vi "nearCamSetExpoureTime.vi"(6 "错误输入（无错误）":errorcluster, 7 "Time/us":dbl, 8 "IMAQdx Session":T1) -> (0 "错误输出":errorcluster, 1 "MaxDBL":dbl, 3 "TimeOut":dbl, 4 "MinDBL":dbl, 5 "IMAQdx Session Out":T1)   [LabVIEW 2018]
uses:
  <vilib>/userdefined/High Color/IMAQdx.ctl
  <resource>/objmgr/imaqdx.rc
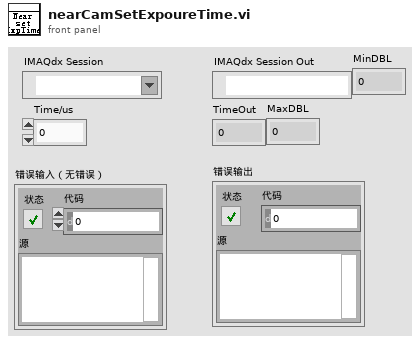
[diagram p1: front panel]
types:
  T1 = typedef "IMAQdx.ctl" = refnum<k21>
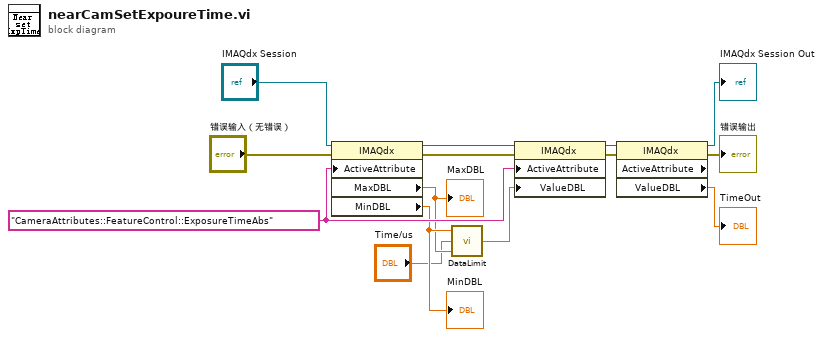
[diagram p0: block diagram]
diagram:
  w13 = "CameraAttributes::FeatureControl::ExposureTimeAbs" ("ActiveAttribute")
  n1 = property class="IMAQdx"(reference="IMAQdx Session", error in="错误输入（无错误）", "ActiveAttribute"=w13) -> (reference out=w14:T1, error out=w9:errorcluster, "MaxDBL"=w11:dbl, "MinDBL"=w12:dbl)
  "MaxDBL" <- w11
  "MinDBL" <- w12
  n2 = call "DataLimit.vi"("Max"=w11, "Data"="Time/us", "Min"=w12) -> ("Data Out"=w10:dbl)  [unwired: 2 in]
  n3 = property class="IMAQdx"(reference=w14, error in=w9, "ActiveAttribute"=w13, "ValueDBL"=w10) -> (reference out=w7:T1, error out=w5:errorcluster)
  n4 = property class="IMAQdx" props=["ActiveAttribute", "ValueDBL"](reference=w7, error in=w5) -> (reference out=→"IMAQdx Session Out":T1, error out=→"错误输出":errorcluster, "ValueDBL"=→"TimeOut":dbl)  [unwired: 1 out]
